vi "Write Setpoint.vi"(8 "error in (no error)":errorcluster, 10 "Setpoint":dbl, 11 "Send New Setpoint in":refnum<class "Send New Setpoint.lvclass">) -> (0 "error out":errorcluster, 3 "Send New Setpoint out":refnum<class "Send New Setpoint.lvclass">)   [LabVIEW 2015, in "Send New Setpoint.lvclass"]
uses:
  Send New Setpoint.lvclass
  Send New Setpoint.lvclass/Send New Setpoint.ctl
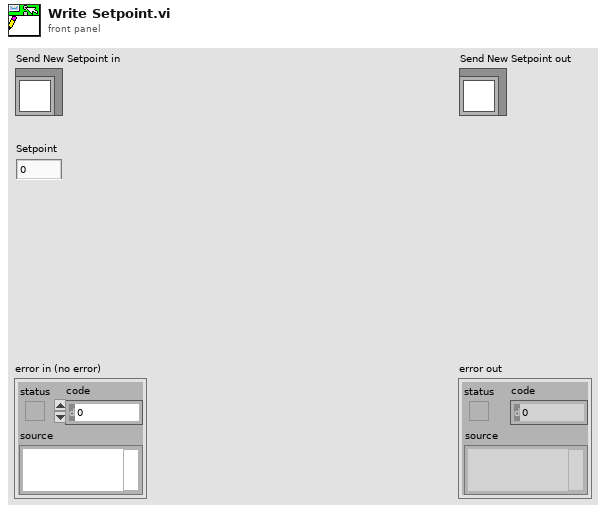
[diagram p1: front panel]
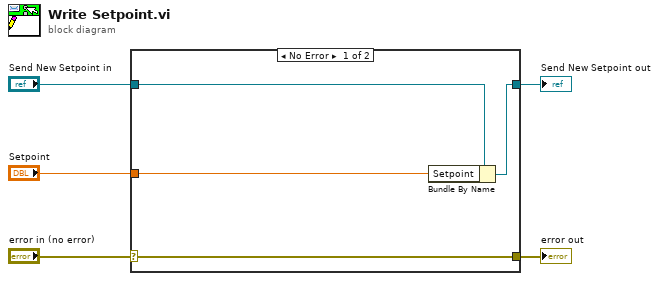
[diagram p0: block diagram]
diagram:
  n1 = case shown="No Error" "error in (no error)" {
    selector: "error in (no error)" -> [w9 w10]
    tunnel: [w9 w10] -> w4
    tunnel: [w7 w11] -> w2
    tunnel: "Send New Setpoint in" -> [w8 w11]
    tunnel: "Setpoint" -> [w6 _]
    frame No Error {
      n2 = Bundle By Name(cluster=w8, "Setpoint"=w6) -> (w7:refnum<class "Send New Setpoint.lvclass">)
    }
    frame Error {
    }
  }
  "error out" <- w4
  "Send New Setpoint out" <- w2
